vi "Dashboard Main.vi"(0 "Dashboard Tab":T1(tab)=enum."Custom") -> ()   [LabVIEW 2015]
uses:
  <vilib>/Utility/miscctls.llb/LVRowAndColumnTypeDef.ctl
  <vilib>/event_ctls.llb/eventvkey.ctl
  <vilib>/Rock Robotics/WPI/Dashboard/WPI_DashboardLogging Global.vi
  <vilib>/Rock Robotics/Network Tables/NT Read Numeric Array.vi
  <vilib>/Utility/config.llb/Write Key (String).vi
  <vilib>/Utility/config.llb/Write Key (I32).vi
  <vilib>/Utility/config.llb/NI_LVConfig.lvlib
panel:
  in  "TCP":refnum<k5>
  in  "Rec Mode":enum32{"Stop", "Record", "Playback"}(radio)
  in  "Vision":u16(ring) items=["Camera Off", "USB Camera SW", "USB Camera HW", "IP Camera"]
  out "Camera IP":string="172.22.11.2"
  out "Image Message":string="Timeout in Camera Communications"
  in  "Select Auto":string(combo)
  out "NT Connection":bool
  in  "Camera Settings":T2={"Frame Rate"=17, "Compression"=30, "Size"=1} {"Frame Rate" scale=1.0..30.0; "Size" items=["640x480", "320x240", "160x120"]}
  out "MotorChart R":cluster{"Numeric":dbl, "Numeric":dbl}(graph)
  out "MotorChart L":T3(graph)={"Numeric"=0.0, "Numeric"=0.0, "Battery V"=12.03125}
  out "MotorSliders R":cluster{"MotorSlide1":dbl, "MotorSlide2":dbl} {"MotorSlide2" scale=-1.0..1.0 scale format="%#_2e"; "MotorSlide1" scale=-1.0..1.0 scale format="%#_2e"}
  out "MotorSliders L":T4={"MotorSlide1"=0.0, "MotorSlide2"=0.0, "MotorSlide4 2"=12.03125} {"MotorSlide4 2" scale=0.0..14.0 scale format="%#_2e"; "MotorSlide2" scale=-1.0..1.0 scale format="%#_2e"; "MotorSlide1" scale=-1.0..1.0 scale format="%#_2e"}
  out "Gyro":dbl(knob) scale=0.0..360.0
  out "JS1 Z":dbl(slide) scale=-1.0..1.0 scale format="%#_2e"
  out "JS1 Graph":cluster{"X":dbl, "Y":dbl}[](graph)
  out "JS1 Buttons":T5
  out "JS2 Z":dbl(slide) scale=-1.0..1.0 scale format="%#_2e"
  out "JS2 Graph":cluster{"X":dbl, "Y":dbl}[](graph)
  out "JS2 Buttons":T5
  out "Mode":T6(ring)=enum."No Code"
  in  "DB Camera Config":bool
  out "fps":dbl format="%#.1g"
  out "Mbps":dbl format="%#.1g"
  out "Mbps LED":bool
  in  "DB/String 9":string
  in  "DB/String 8":string
  in  "DB/String 7":string
  in  "DB/String 6":string
  in  "DB/String 5":string
  in  "DB/String 4":string
  in  "DB/String 3":string
  in  "DB/String 2":string
  in  "DB/String 1":string
  in  "DB/String 0":string
  in  "DB/Slider 0":dbl(slide) scale=0.0..5.0
  in  "DB/Slider 1":dbl(slide) scale=0.0..5.0
  in  "DB/Slider 2":dbl(slide) scale=0.0..5.0
  in  "DB/Slider 3":dbl(slide) scale=0.0..5.0
  out "DB/LED 3":bool
  out "DB/LED 2":bool
  out "DB/LED 1":bool
  out "DB/LED 0":bool
  in  "DB/Button 3":bool
  in  "DB/Button 2":bool
  in  "DB/Button 1":bool
  in  "DB/Button 0":bool caption="New Name"
  in  "Left":bool
  out "Dist":dbl
  in  "Man_Cam":dbl
  out "Waveform Chart":cluster{"Numeric":dbl, "Numeric":dbl}(graph)
  in  "Shoot_Auto":bool
  in  "Auto":string(combo)
  in  "Delay_Auto":dbl(slide) scale=0.0..5.0
  in  "DB/MAO_Shooter":dbl
  in  "DB/Ramp_Rate":dbl=1.75
  in  "DB/FF_Gain":dbl=0.13
  in  "DB/I_Gain":dbl=1.0
  in  "DB/D_Gain":dbl
  in  "DB/P_Gain":dbl=0.03
  out "Angle_Error":dbl
  in  "En_Manual_Cam":bool
  in  "DB/Close":dbl=20.0
  in  "DB/Far_Cam":dbl=240.0
  in  "DB/Pitch_Dist":dbl=130.0
  in  "Right":bool
  in  "Test Slider":dbl(slide) scale=0.0..100.0 scale format="%#_3g"
  in  "On/Off":bool caption="Solenoid"
  in  "Test Name":u16(ring) items=["Select the test to run..."]
  in  "Test Tree":string(tree)
  in  "Motor":cluster{"Value":dbl, "Enable":bool} {"Value" scale=-1.0..1.0 scale format="%#_3g"}
  out "Progress":T7 {"Test Progress" scale=0.0..100.0}
  in  "Rev/Fwd":cluster{"Forward":bool, "Reverse":bool}
  in  "Test Ring":u16(ring) items=["Monochrome", "Color"]
  out "Cmd Status":string
  in  "Execute Command":bool
  in  "Command Params":string[][](table)
  in  "Command Selection":i32(listbox)
  in  "CheckList":i32(listbox)
  out "Tree":string(tree)
  out "Camera Image":T8(plugin-control)
  out "Background":bool
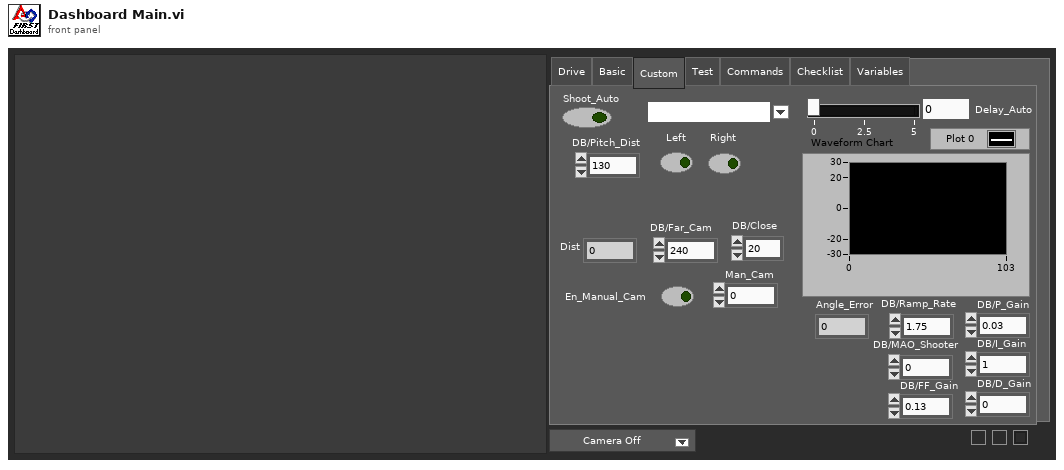
[diagram p1: front panel]
types:
  T1 = enum32{"Drive", "Basic", "Custom", "Test", "Commands", "Checklist", "Variables"}
  T2 = cluster{"Frame Rate":i32, "Compression":i32, "Size":u16}
  T3 = cluster{"Numeric":dbl, "Numeric":dbl, "Battery V":dbl}
  T4 = cluster{"MotorSlide1":dbl, "MotorSlide2":dbl, "MotorSlide4 2":dbl}
  T5 = cluster{bool, bool, bool, bool, bool, bool, bool, bool, bool, bool, bool, bool}
  T6 = enum8{"Tele-Op Disabled", "Tele-Op Enabled", "Auto Disabled", "Auto Enabled", "Test Disabled", "Test Enabled", "Disconnected", "No Code", "E-Stop"}
  T7 = cluster{"Test Progress":u8, "Test Progress Text":string}
  T8 = typedef "IMAQ Image.ctl" = refnum<image>
  T9 = cluster{"IDs":cluster{"RPC field ID":u16, "Unique ID":u16}, "String":string}
  T10 = enum32{"Drive", "Basic", "Custom", "Test", "Checklist", "Variables"}
  T11 = typedef "Image Type" = u32
  T12 = cluster{"Camera Image":refnum<vi>, "Dashboard Tab":refnum<vi>, "Background":refnum<vi>, "Vision":refnum<vi>, "Rec Mode":refnum<vi>, "Test Slider":refnum<vi>, "On/Off ":refnum<vi>, "Test Ring":refnum<vi>, "Rev/Fwd":refnum<vi>, "Test Name":refnum<vi>, "Motor":refnum<vi>, "Progress":refnum<vi>, "CheckList":refnum<vi>, "Tree":refnum<vi>, "Test Tree":refnum<vi>, "Command Params":refnum<vi>, "Command Selection":refnum<vi>, "Execute Command":refnum<vi>, "Cmd Status":refnum<vi>}
  T13 = cluster{"Error Strings":string, "Disable Counts":cluster{u16, u16}, "Rail Faults":cluster{u16, u16, u16}, "Robot IP":string, "DB Mode":u8, "Event Info":cluster{"Name":string, "Type":u8, "Number":u16, "Replay":u8}, "Camera Addr":string}
  T14 = cluster{"Storage":cluster{"Disk Free":u64, "RAM Block":u32, "RAM free":u32}, "CPU Utilization":cluster{"CPU % ISR":sgl, "CPU % Time Crit":sgl, "CPU % Timed Str":sgl, "CPU % High":sgl, "CPU % Above":sgl, "CPU % Normal":sgl, "CPU % Low":sgl}, "CAN":cluster{"% Bus Utilization":sgl, "Bus Off Cnt":u32, "TX_FIFO Full Cnt":u32, "Receive Error Cnt":u8, "Transmit Error Cnt":u8}, "HID":cluster{"HID Outputs":u32, "Rumble Low":u16, "Rumble High":u16}[]}
  T15 = cluster{"Status bits":cluster{"Test Mode":bool, "Autonomous":bool, "Enabled":bool, "Code Start":bool, "Brownout":bool, "Reserved 2":bool, "Reserved 3":bool, "E-Stop":bool}, "Code Trace":cluster{"Disabled":bool, "TeleOp":bool, "Auto":bool, "Test":bool}, "Controller Type":enum16{"unknown", "cRIO", "roboRio"}, "Code?":enum16{"unknown", "noCode", "code"}, "Battery V":dbl}
  T16 = cluster{"Control Bits":cluster{"TestMode":bool, "Autonomous":bool, "Enabled":bool, "FMS Present":bool, bool, bool, bool, "E-Stop":bool}, "Team Station ":u8, "Countdown":sgl, "Joystick Values":cluster{"Axes":dbl[], "Buttons":bool[], "POVs":i16[]}[]}
  T17 = cluster{"Axes":dbl[], "Buttons":bool[], "POVs":i16[]}[]
  T18 = cluster{"Axes":dbl[], "Buttons":bool[], "POVs":i16[]}
  T19 = cluster{"Buttons[0]":bool, "Buttons[1]":bool, "Buttons[2]":bool, "Buttons[3]":bool, "Buttons[4]":bool, "Buttons[5]":bool, "Buttons[6]":bool, "Buttons[7]":bool, "Buttons[8]":bool, "Buttons[9]":bool, "Buttons[10]":bool, "Buttons[11]":bool}
  T20 = typedef "NI_LVConfig.lvlib/Config Data RefNum.ctl" = refnum<k1>
  T21 = cluster{"Operation":enum16{"Update", "Clear"}, "Color Box":u32}[]
  T22 = typedef "eventvkey.ctl" = enum16{"ASCII", "Enter", "Return", "Shift", "Ctrl", "Alt", "Cmd", "Opt", "Caps", "NumLock", "Clear", "Break", "Up", "Down", "Left", "Right", "Insert", "Delete", "Home", "End", "PageUp", "PageDown", "Escape", "Help", "Pause", "ScrollLock", "F1", "F2", "F3", "F4", "F5", "F6", "F7", "F8", "F9", "F10", "F11", "F12", "F13", "F14", "F15", "F16", "F17", "F18", "F19", "F20", "F21", "F22", "F23", "F24", "Play", "VolumeUp", "VolumeDown", "Mute", "Two Byte Char"}
  T23 = cluster{"Image Size":bool, "Image Type":bool, "Pixel Value":bool, "ROI Information":bool, "Zoom Factor":bool}
  T24 = enum8{"Enabled", "Disabled", "Disabled and Grayed Out"}
  T25 = cluster{"Operation":enum16{"Update", "Clear"}, "Color Box":u32}
  T26 = typedef "LVRowAndColumnTypeDef.ctl" = cluster{"Row":i32, "Column":i32}
  T27 = cluster{"Shift":bool, "Ctrl":bool, "Alt":bool, "Cmd":bool, "Opt":bool}
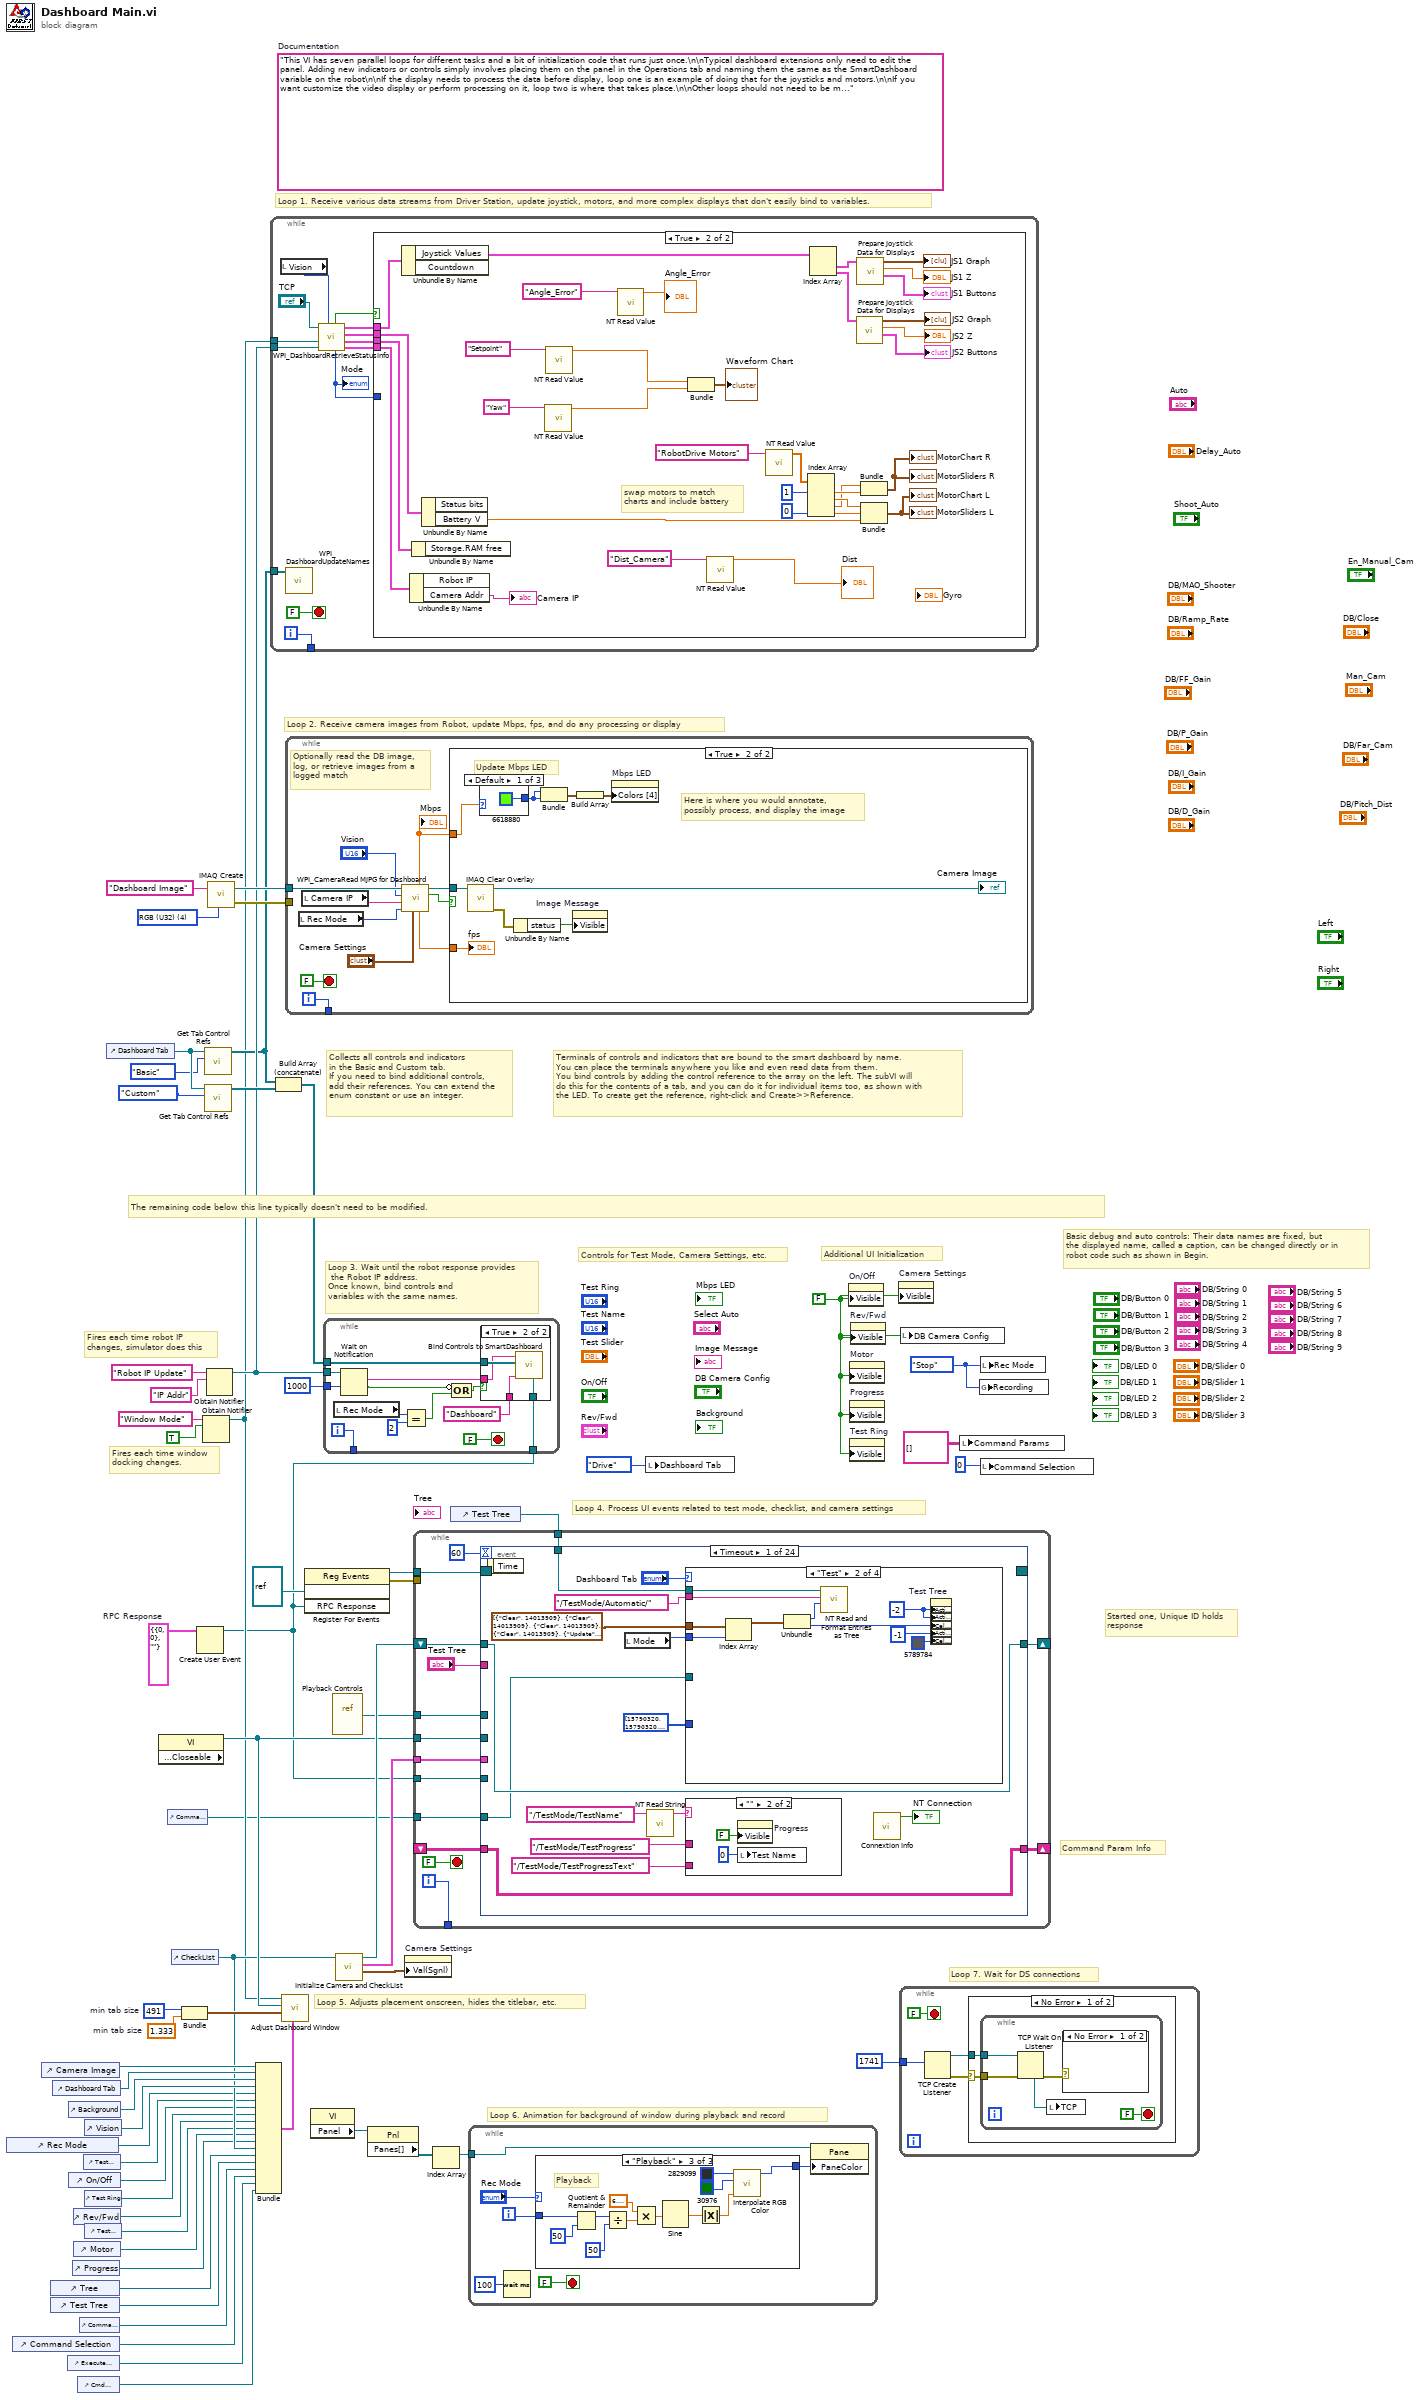
[diagram p0: block diagram]
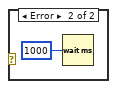
[diagram p2: hidden frame]
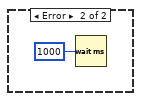
[diagram p3: hidden frame]
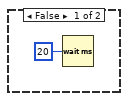
[diagram p4: hidden frame]
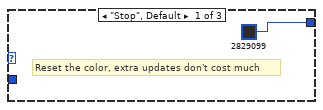
[diagram p5: hidden frame]
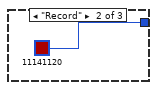
[diagram p6: hidden frame]
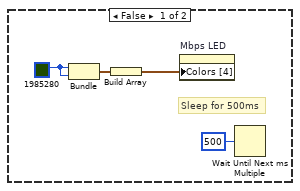
[diagram p8: hidden frame]
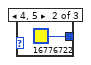
[diagram p9: hidden frame]
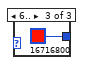
[diagram p10: hidden frame]
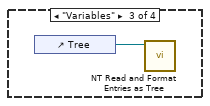
[diagram p12: hidden frame]
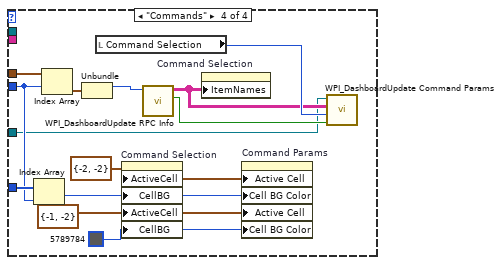
[diagram p13: hidden frame]
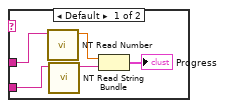
[diagram p14: hidden frame]
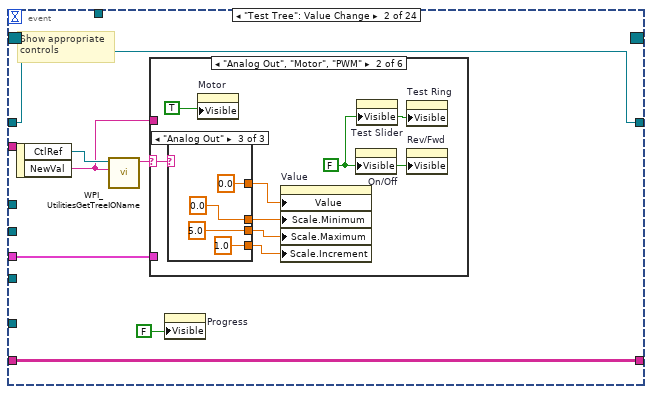
[diagram p15: hidden frame]
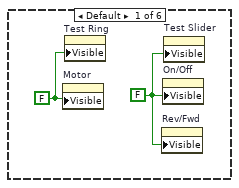
[diagram p16: hidden frame]
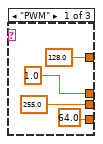
[diagram p17: hidden frame]
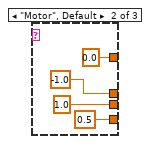
[diagram p18: hidden frame]
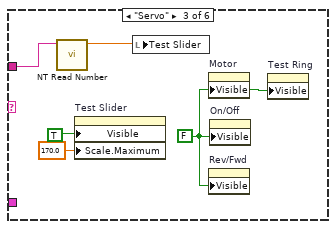
[diagram p19: hidden frame]
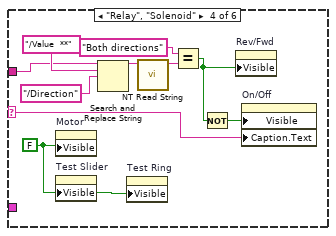
[diagram p20: hidden frame]
diagram:
  w7 = T9 {"IDs"={"RPC field ID"=0, "Unique ID"=0}, "String"=""}  # RPC Response
  w33 = 491  # min tab size
  w32 = 1.333  # min tab size
  w41 = enum32{"Stop", "Record", "Playback"}."Stop" ("Rec Mode")
  w15 = FALSE ("Visible")
  (unwired) "This VI has seven parallel loops for different tasks and a bit of initialization code that runs just once.\n\nTypical dashboard extensions only need to edit the panel. Adding new indicators or controls simply involves placing them on the panel in the Operations tab and naming them the same as the SmartDashboard variable on the robot\n\nIf the display needs to process the data before display, loop one is an example of doing that for the joysticks and motors.\n\nIf you want customize the video display or perform processing on it, loop two is where that takes place.\n\nOther loops should not need to be modified. They are pretty standard, and document the task they perform."  # Documentation
  w61 = T11 4 items=["Grayscale (U8)", "Grayscale (I16)", "Grayscale (SGL)", "Complex (CSG)", "RGB (U32)", "HSL (U32)", "RGB (U64)"] ("Image Type")
  # "Command Param Info"
  # "Started one, Unique ID holds\nresponse"
  # "Loop 7. Wait for DS connections"
  # "Basic debug and auto controls: Their data names are fixed, but\nthe displayed name, called a caption, can be changed directly or in\nrobot code such as shown in Begin."
  # "Controls for Test Mode, Camera Settings, etc."
  # "Additional UI Initialization"
  # "Loop 6. Animation for background of window during playback and record"
  # "Fires each time robot IP\nchanges, simulator does this"
  # "Fires each time window\ndocking changes."
  # "Collects all controls and indicators\nin the Basic and Custom tab.\nIf you need to bind additional controls,\nadd their references. You can extend the\nenum constant or use an integer."
  # "The remaining code below this line typically doesn't need to be modified."
  # "Loop 4. Process UI events related to test mode, checklist, and camera settings"
  # "Terminals of controls and indicators that are bound to the smart dashboard by name.\nYou can place the terminals anywhere you like and even read data from them.\nYou bind controls by adding the control reference to the array on the left. The subVI will\ndo this for the contents of a tab, and you can do it for individual items too, as shown with\nthe LED. To create get the reference, right-click and Create>>Reference."
  # "Loop 3. Wait until the robot response provides\n the Robot IP address.\nOnce known, bind controls and\nvariables with the same names."
  # "Loop 5. Adjusts placement onscreen, hides the titlebar, etc."
  # "Loop 1. Receive various data streams from Driver Station, update joystick, motors, and more complex displays that don't easily bind to variables."
  # "Loop 2. Receive camera images from Robot, update Mbps, fps, and do any processing or display"
  n1 = control-ref of="Rec Mode"() -> (w21:refnum<vi>)
  n2 = control-ref of="Command Selection"() -> (w6:refnum<vi>)
  n3 = control-ref of="Camera Image"() -> (w36:refnum<vi>)
  n4 = control-ref of="Tree"() -> (w25:refnum<vi>)
  n5 = control-ref of="Test Tree"() -> (w24:refnum<vi>)
  n6 = control-ref of="Dashboard Tab"() -> (w35:refnum<vi>)
  n7 = control-ref of="Execute Command"() -> (w8:refnum<vi>)
  n8 = control-ref of="Background"() -> (w30:refnum<vi>)
  n9 = control-ref of="On/Off"() -> (w19:refnum<vi>)
  n10 = control-ref of="Progress"() -> (w16:refnum<vi>)
  n11 = control-ref of="Rev/Fwd"() -> (w17:refnum<vi>)
  n12 = control-ref of="Motor"() -> (w22:refnum<vi>)
  n13 = control-ref of="Cmd Status"() -> (w2:refnum<vi>)
  n14 = control-ref of="Command Params"() -> (w9:refnum<vi>)
  n15 = control-ref of="Test Slider"() -> (w20:refnum<vi>)
  n16 = control-ref of="Vision"() -> (w34:refnum<vi>)
  n17 = control-ref of="Test Ring"() -> (w18:refnum<vi>)
  n18 = control-ref of="Test Name"() -> (w23:refnum<vi>)
  n19 = control-ref of="Dashboard Tab"() -> (w39:refnum<vi>)
  n20 = property class="VI" props=["Front Panel.Closeable"]() -> (reference out=w40:refnum<vi>)  [unwired: 2 in, 2 out]
  n21 = control-ref of="Command Params"() -> (w1:refnum<vi>)
  n22 = control-ref of="CheckList"() -> (w26:refnum<vi>)
  n23 = Bundle("min tab size"=w33, "min tab size"=w32) -> (w31:cluster{"min tab size":i32, "min tab size":dbl})  [unwired: 1 in]
  n24 = Create User Event(user event datatype=w7) -> (user event=w3:refnum<user-event>)  [unwired: 1 in, 1 out]
  n25 = Obtain Notifier(name (unnamed)="Window Mode", notification data type=TRUE) -> (notifier out=w12:refnum<notifier>)  [unwired: 2 in, 2 out]
  n26 = call <vilib>:"Get Tab Control Refs.vi"("Page Index"=T10."Basic" ("Dashboard Tab"), "TabControl in"=w39) -> ("ControlsOnPage"=w13:refnum<vi>[])  [unwired: 9 in]
  n27 = call <vilib>:"Get Tab Control Refs.vi"("Page Index"=T10."Custom" ("Dashboard Tab"), "TabControl in"=w39) -> ("ControlsOnPage"=w38:refnum<vi>[])  [unwired: 9 in]
  n28 = Obtain Notifier(name (unnamed)="Robot IP Update", notification data type="IP Addr" ("name (unnamed)")) -> (notifier out=w14:refnum<notifier>)  [unwired: 2 in, 2 out]
  n29 = call "IMAQ Create"("Image Name"="Dashboard Image", "Image Type"=w61) -> ("New Image"=w59:T8, "error out"=w58:errorcluster)  [unwired: 2 in, 1 out]
  n30 = Bundle("Camera Image"=w36, "Dashboard Tab"=w35, "Background"=w30, "Vision"=w34, "Rec Mode"=w21, "Test Slider"=w20, "On/Off"=w19, "Test Ring"=w18, "Rev/Fwd"=w17, "Test Name"=w23, "Motor"=w22, "Progress"=w16, "CheckList"=w26, "Tree"=w25, "Test Tree"=w24, "Command Params"=w9, "Command Selection"=w6, "Execute Command"=w8, "Cmd Status"=w2) -> (w27:T12)  [unwired: 1 in]
  n31 = while {
    tunnel: [w73] -> _
    tunnel: w14 -> [w67]
    tunnel: w13 -> [w66]
    tunnel: w12 -> [w62]
    i -> [w73]
    stop <- FALSE stop-if-true
    n32 = local read "Vision"() -> (w64:u16)
    n33 = call <vilib>:"WPI_DashboardUpdateNames.vi"("Controls on Tab"=w66) -> ()  [unwired: 11 in]
    n34 = call <vilib>:"WPI_DashboardRetrieveStatusInfo.vi"("Vision"=w64, "Binding Refnum"=w67, "Window Mode Notifier"=w62, "TCP Cnx"="TCP") -> ("Power and Errors"=w68:T13, "Robot Metrics"=w71:T14, "Status Info"=w72:T15, "Control Info"=w69:T16, "Robot Mode"=w65:T6, "Process?"=w70:bool)  [unwired: 2 in]
    "Mode" <- w65
    n35 = case shown="True" w70 {
      tunnel: w72 -> [_ w109]
      tunnel: w71 -> [_ w108]
      tunnel: w69 -> [_ w107]
      tunnel: w68 -> [_ w106]
      tunnel: w65 -> [_ _]
      frame False {
        n36 = Wait (ms)(milliseconds to wait=u32 20) -> ()  [unwired: 1 out]
      }
      frame True {
        # "swap motors to match\ncharts and include battery"
        n37 = Unbundle By Name(w107) -> ("Joystick Values"=w96:T17)  [unwired: 1 out]
        n38 = Unbundle By Name(w106) -> ("Camera Addr"=→"Camera IP":string)  [unwired: 1 out]
        n39 = Unbundle By Name(w108) -> ()  [unwired: 1 out]
        n40 = Unbundle By Name(w109) -> ("Battery V"=w97:dbl)  [unwired: 1 out]
        n41 = call-poly <vilib>:"NT Read Value.vi"("Name"="Yaw") -> ("Numeric"=w79:dbl)  [unwired: 9 in, 1 out]
        n42 = call-poly <vilib>:"NT Read Value.vi"("Name"="Setpoint") -> ("Numeric"=w80:dbl)  [unwired: 9 in, 1 out]
        n43 = call-poly <vilib>:"NT Read Value.vi"("Name"="Angle_Error") -> ("Numeric"=→"Angle_Error":dbl)  [unwired: 9 in, 1 out]
        n44 = Bundle("Numeric"=w80, "Numeric"=w79) -> (→"Waveform Chart":cluster{"Numeric":dbl, "Numeric":dbl})  [unwired: 1 in]
        n45 = call-poly <vilib>:"NT Read Value.vi"("Name"="Dist_Camera") -> ("Numeric"=→"Dist":dbl)  [unwired: 9 in, 1 out]
        n46 = call-poly <vilib>:"NT Read Value.vi"("Name"="RobotDrive Motors") -> ("Numeric Array"=w85:dbl[])  [unwired: 9 in, 1 out]
        n47 = Index Array(array=w85, index #1=1, index #4=0) -> (element #1=w101:dbl, element #2=w102:dbl, element #3=w100:dbl, element #4=w105:dbl)  [unwired: 2 in]
        n48 = Index Array(array=w96) -> (element #1=w95:T18, element #2=w90:T18)  [unwired: 2 in]
        n49 = call "Prepare Joystick Data for Displays.vi"("Joystick Values"=w90) -> ("Buttons"=→"JS2 Buttons":T19, "Z Axis"=→"JS2 Z":dbl, "Cartesian Data"=→"JS2 Graph":cluster{"X axis":dbl, "X axis":dbl}[])  [unwired: 8 in]
        n50 = call "Prepare Joystick Data for Displays.vi"("Joystick Values"=w95) -> ("Buttons"=→"JS1 Buttons":T19, "Z Axis"=→"JS1 Z":dbl, "Cartesian Data"=→"JS1 Graph":cluster{"X axis":dbl, "X axis":dbl}[])  [unwired: 8 in]
        n51 = Bundle("Numeric"=w100, "Numeric"=w101) -> (→"MotorChart R" →"MotorSliders R":cluster{"Numeric":dbl, "Numeric":dbl})  [unwired: 1 in]
        n52 = Bundle("Numeric"=w102, "Numeric"=w105, "Battery V"=w97) -> (→"MotorChart L" →"MotorSliders L":T3)  [unwired: 1 in]
      }
    }
  }
  n53 = Build Array (concatenate)(w13, w38) -> (w37:refnum<vi>[])
  n54 = call "Adjust Dashboard Window.vi"("Sizing Refnums"=w27, "Size Constraints"=w31, "VI"=w40, "WIn Mode"=w12) -> ()  [unwired: 8 in]
  n55 = while {
    tunnel: w59 -> [w118]
    tunnel: w58 -> [_]
    tunnel: [w119] -> _
    i -> [w119]
    stop <- FALSE stop-if-true
    # "Optionally read the DB image,\nlog, or retrieve images from a\nlogged match"
    n56 = local read "Rec Mode"() -> (w113:enum32{"Stop", "Record", "Playback"})
    n57 = local read "Camera IP"() -> (w111:string)
    n58 = call <vilib>:"WPI_CameraRead MJPG for Dashboard.vi"("Camera Settings"="Camera Settings", "Rec Mode"=w113, "Camera IP"=w111, "Camera Mode"="Vision", "Refnum in"=w118) -> ("Active"=w116:bool, "Refnum out"=w117:T8, "FPS"=w115:dbl, "Bandwidth (Mbps)"=w110:dbl)  [unwired: 3 in]
    "Mbps" <- w110
    n59 = case shown="True" w116 {
      tunnel: w117 -> [_ w128]
      tunnel: w110 -> [_ w127]
      tunnel: w115 -> [_ w125]
      frame False {
        w121 = u32 1985280 ("Color Box")
        # "Sleep for 500ms"
        n60 = Bundle("Color Box"=w121, "Color Box"=w121) -> (w123:cluster{"Color Box":u32, "Color Box":u32})  [unwired: 1 out]
        n61 = Build Array(w123) -> (w122:cluster{"Color Box":u32, "Color Box":u32}[])
        n62 = property on="Mbps LED" class="Bool (strict)"("Colors [4]"=w122) -> ()  [unwired: 2 in, 2 out]
        n63 = Wait Until Next ms Multiple(millisecond multiple=u32 500) -> ()  [unwired: 1 out]
      }
      frame True {
        # "Here is where you would annotate,\npossibly process, and display the image"
        # "Update Mbps LED"
        n64 = call "IMAQ Clear Overlay"("Image"=w128) -> ("error out"=w132:errorcluster, "Image Out"=→"Camera Image":T8)  [unwired: 2 in, 7 out]
        n65 = case shown="Default" w127 {
          tunnel: [u32 6618880 ("Color Box") u32 16776722 ("Color Box") u32 16716800 ("Color Box")] -> w129
          frame Default {
          }
          frame 4, 5 {
          }
          frame 6.. {
          }
        }
        n66 = Unbundle By Name(w132) -> ("status"=w133:bool)
        n67 = Bundle("Color Box"=w129, "Color Box"=w129) -> (w131:cluster{"Color Box":u32, "Color Box":u32})  [unwired: 1 out]
        n68 = property on="Image Message" class="Str"("Visible"=w133) -> ()  [unwired: 2 in, 2 out]
        n69 = Build Array(w131) -> (w130:cluster{"Color Box":u32, "Color Box":u32}[])
        n70 = property on="Mbps LED" class="Bool (strict)"("Colors [4]"=w130) -> ()  [unwired: 2 in, 2 out]
        "fps" <- w125
      }
    }
  }
  n71 = register-events(refnum<vi> refnum, w3) -> (reference out=w45:refnum<event-registration>, error out=w44:errorcluster)  [unwired: 2 in]
  n72 = property class="VI"() -> ("Panel"=w48:refnum<vi>)  [unwired: 2 in, 2 out]
  n73 = while {
    tunnel: w37 -> [w149]
    tunnel: w14 -> [w147]
    tunnel: [w145] -> _
    tunnel: u32 1000 ("milliseconds to wait") -> [w144]
    tunnel: w3 -> [w137]
    i -> [w145]
    stop <- FALSE stop-if-true
    n74 = local read "Rec Mode"() -> (w140:enum32{"Stop", "Record", "Playback"})
    n75 = Wait on Notification(notifier=w147, timeout in ms (-1)=w144) -> (notification=w146:string, timed out?=w142:bool)  [unwired: 2 in, 2 out]
    n76 = Equal?(x=w140, y=u16 2 ("Rec Mode")) -> (x = y?=w141:bool)
    n77 = Compound Arithmetic op=OR(invert w142, w141) -> (w143:bool)
    n78 = case shown="True" w143 {
      tunnel: w149 -> [_ w153]
      tunnel: w146 -> [_ w152]
      tunnel: "Dashboard" -> [_ w151]
      tunnel: w137 -> [_ w150]
      frame False {
      }
      frame True {
        n79 = call <vilib>:"Bind Controls to SmartDashboard.vi"("RPC ref"=w150, "Client Name"=w151, "Bound Control Refs"=w153, "Server IP Address"=w152) -> ()  [unwired: 8 in]
      }
    }
  }
  n80 = vi-ref "Playback Controls.vi"() -> (w46:refnum<vi>)
  n81 = call "Initialize Camera and CheckList.vi"("ListBox in"=w26) -> ("Cluster"=w52:cluster{"value":i32, "value":i32, "index":i32}, "Array"=w53:cluster{string[]}[], "File Refnum"=w51:T20)  [unwired: 8 in]
  n82 = property class="Pnl"(reference=w48) -> ("Panes[]"=w49:refnum<vi>[])  [unwired: 1 in, 2 out]
  n83 = property on="Camera Settings" class="Clust (strict)"("Val(Sgnl)"=w52) -> ()  [unwired: 2 in, 2 out]
  n84 = Index Array(array=w49) -> (element=w47:refnum<vi>)  [unwired: 1 in]
  n85 = control-ref of="Test Tree"() -> (w50:refnum<vi>)
  n86 = while {
    tunnel: w53 -> [w165]
    shift-right: [w164] -> _
    shift-left: w51 -> [w163]
    tunnel: [w162] -> _
    tunnel: w50 -> [w161]
    tunnel: w46 -> [w160]
    tunnel: w45 -> [w159]
    tunnel: w44 -> [_]
    tunnel: w40 -> [w158]
    tunnel: w3 -> [w157]
    tunnel: w1 -> [w156]
    shift-right: [w155] -> _
    shift-left: _ -> [w154]
    i -> [w162]
    stop <- FALSE stop-if-true
    n87 = event shown="[0] Timeout" {
      selector: w159 -> [_ _ _ _ _ _ _ _ _ _ _ _ _ _ _ _ _ _ _ _ _ _ _ _]
      dyn-events: [_ _ _ _ _ _ _ _ _ _ _ _ _ _ _ _ _ _ w474 _ _ _ _ _] -> _
      timeout: u32 60 ("milliseconds to wait") -> [_ _ _ _ _ _ _ _ _ _ _ _ _ _ _ _ _ _ _ _ _ _ _ _]
      tunnel: w161 -> [w178 _ _ _ _ _ _ _ _ _ _ _ _ _ _ _ _ _ _ _ _ _ _ _]
      tunnel: "Test Tree" -> [_ _ _ _ _ _ _ _ _ _ _ _ _ w437 w446 w449 w454 w463 _ _ _ _ _ _]
      tunnel: w165 -> [_ w216 _ _ _ _ _ _ _ _ _ w399 w430 _ _ _ _ _ _ _ _ _ _ _]
      tunnel: [w175 w215 w319 w325 w335 w339 w345 w357 w365 w371 w384 w398 w423 w436 w444 w448 w453 w462 w476 w492 w494 w502 w513 w518] -> w164
      tunnel: w163 -> [w175 w215 w319 w325 w335 w339 w345 w357 w365 w371 w384 w397 w423 w436 w444 w448 w453 w462 w476 w492 w494 w502 w513 w518]
      tunnel: w160 -> [_ _ _ _ _ _ _ _ _ _ _ _ _ _ _ _ _ _ w477 _ w497 _ _ _]
      tunnel: w158 -> [_ _ _ _ _ _ _ _ _ _ _ _ _ _ _ _ _ _ w472 _ _ _ _ _]
      tunnel: w157 -> [_ _ _ _ _ _ _ _ _ _ _ _ _ _ _ _ _ _ w468 _ _ _ _ _]
      tunnel: w156 -> [w170 _ _ _ _ _ w343 _ _ _ _ _ _ _ _ _ _ _ _ _ _ _ _ _]
      tunnel: [w169 w214 w318 w324 w334 w340 w341 w351 w362 w370 w383 w396 w422 w435 w443 w447 w452 w461 w467 w490 w493 w498 w506 w519] -> w155
      tunnel: w154 -> [w169 w214 w318 w324 w334 w340 w341 _ _ w370 w383 w396 w422 w435 w443 w447 w452 w461 w467 w490 w493 w498 w506 w519]
      event Timeout {
        n88 = event-data() -> ()  [unwired: 1 in, 1 out]
        n89 = local read "Mode"() -> (w172:T6)
        n90 = call <vilib>:"NT Read String.vi"("Name"="/TestMode/TestName") -> ("String"=w181:string)  [unwired: 9 in, 1 out]
        n91 = case shown="\"Test\"" "Dashboard Tab" {
          tunnel: w178 -> [_ w192 _ _]
          tunnel: "/TestMode/Automatic/" ("Name Pattern") -> [_ w191 _ _]
          tunnel: T21 [{"Operation"=enum."Clear", "Color Box"=14013909}, {"Operation"=enum."Clear", "Color Box"=14013909}, {"Operation"=enum."Clear", "Color Box"=14013909}, {"Operation"=enum."Clear", "Color Box"=14013909}, {"Operation"=enum."Update", "Color Box"=14013909}, {"Operation"=enum."Update", "Color Box"=16777215}, {"Operation"=enum."Clear", "Color Box"=14013909}, {"Operation"=enum."Clear", "Color Box"=14013909}, {"Operation"=enum."Clear", "Color Box"=14013909}] -> [_ w184 _ w201]
          tunnel: w172 -> [_ w183 _ w200]
          tunnel: u32[] [15790320, 15790320, 15790320, 15790320, 16777215, 16777215, 15790320, 15790320, 15790320] -> [_ _ _ w206]
          tunnel: w170 -> [_ _ _ w194]
          frame "Custom", Default {
          }
          frame "Test" {
            w190 = -2 ("Active Item:Row Number")
            n92 = Index Array(array=w184, index=w183) -> (element=w185:T25)
            n93 = Unbundle(w185) -> ("Operation"=w186:enum16{"Update", "Clear"}, "Color Box"=w187:u32)
            n94 = call <vilib>:"NT Read and Format Entries as Tree.vi"("Operation"=w186, "Name Pattern"=w191, "Tree Refnum"=w192) -> ()  [unwired: 7 in, 2 out]
            n95 = property on="Test Tree" class="Tree (strict)"("Active Item Row Number"=w190, "ActiveColNum"=w190, "CellBG"=w187, "Active Item Row Number"=-1 ("Active Item:Row Number"), "CellBG"=u32 5789784 ("Color Box")) -> ()  [unwired: 2 in, 2 out]
          }
          frame "Variables" {
            n96 = control-ref of="Tree"() -> (w193:refnum<vi>)
            n97 = call <vilib>:"NT Read and Format Entries as Tree.vi"("Tree Refnum"=w193) -> ()  [unwired: 9 in, 2 out]
          }
          frame "Commands" {
            w202 = u32 5789784 ("Color Box")
            w203 = T26 {"Row"=-1, "Column"=-2} ("Active Cell:Active Cell")
            w205 = T26 {"Row"=-2, "Column"=-2} ("Active Cell:Active Cell")
            n98 = Index Array(array=w206, index=w200) -> (element=w204:u32)
            n99 = Index Array(array=w201, index=w200) -> (element=w199:T25)
            n100 = Unbundle(w199) -> ("Operation"=w198:enum16{"Update", "Clear"})  [unwired: 1 out]
            n101 = local read "Command Selection"() -> (w197:i32)
            n102 = property on="Command Selection" class="MCListbox (strict)"("ActiveCell"=w205, "CellBG"=w204, "ActiveCell"=w203, "CellBG"=w202) -> ()  [unwired: 2 in, 2 out]
            n103 = call <vilib>:"WPI_DashboardUpdate RPC Info.vi"("Operation"=w198) -> ("update"=w196:bool, "commands"=w195:string[][])  [unwired: 9 in]
            n104 = property on="Command Selection" class="MCListbox (strict)"("ItemNames"=w195) -> ()  [unwired: 2 in, 2 out]
            n105 = property on="Command Params" class="Tbl (strict)"("Active Cell"=w205, "Cell BG Color"=w204, "Active Cell"=w203, "Cell BG Color"=w202) -> ()  [unwired: 2 in, 2 out]
            n106 = call <vilib>:"WPI_DashboardUpdate Command Params.vi"("Update"=w196, "NewVal"=w197, "Commands"=w195, "Param Tbl"=w194) -> ()  [unwired: 7 in, 1 out]
          }
        }
        n107 = case shown="\"\"" w181 {
          tunnel: "/TestMode/TestProgress" ("Name") -> [w208 _]
          tunnel: "/TestMode/TestProgressText" ("Name") -> [w207 _]
          frame Default {
            n108 = call <vilib>:"NT Read Number.vi"("Name"=w208) -> ("Numeric"=w209:dbl)  [unwired: 9 in, 1 out]
            n109 = call <vilib>:"NT Read String.vi"("Name"=w207) -> ("String"=w210:string)  [unwired: 9 in, 1 out]
            n110 = Bundle("Numeric"=w209, "String"=w210) -> (→"Progress":cluster{"Numeric":dbl, "String":string})  [unwired: 1 in]
          }
          frame "" {
            n111 = property on="Progress" class="Clust (strict)"("Visible"=FALSE) -> ()  [unwired: 2 in, 2 out]
            n112 = local write "Test Name"(u16 0) -> ()
          }
        }
        n113 = call <vilib>:"Connextion Info.vi"() -> ("Connected"=→"NT Connection":bool)  [unwired: 10 in, 1 out]
      }
      event "Test Tree": Value Change {
        # "Show appropriate\ncontrols"
        n114 = event-data() -> ("CtlRef"=w219:refnum<vi>, "NewVal"=w217:string)  [unwired: 1 in]
        n115 = call <vilib>:"WPI_UtilitiesGetTreeIOName.vi"("NewVal"=w217, "TreeControl in"=w219) -> ("I/O Name"=w220:string)  [unwired: 9 in]
        n116 = case shown="\"Analog Out\", \"Motor\", \"PWM\"" w220 {
          selector: w220 -> [_ w227 _ w249 w258 _]
          tunnel: w217 -> [_ _ w246 w248 _ w265]
          tunnel: w216 -> [_ _ _ _ _ w264]
          frame Default {
            w222 = FALSE ("Visible")
            w221 = FALSE ("Visible")
            n117 = property on="Motor" class="Clust (strict)"("Visible"=w221) -> ()  [unwired: 2 in, 2 out]
            n118 = property on="Test Ring" class="Ring (strict)"("Visible"=w221) -> ()  [unwired: 2 in, 2 out]
            n119 = property on="Rev/Fwd" class="Clust (strict)"("Visible"=w222) -> ()  [unwired: 2 in, 2 out]
            n120 = property on="On/Off" class="Bool (strict)"("Visible"=w222) -> ()  [unwired: 2 in, 2 out]
            n121 = property on="Test Slider" class="Slide (strict)"("Visible"=w222) -> ()  [unwired: 2 in, 2 out]
          }
          frame "Analog Out", "Motor", "PWM" {
            w228 = FALSE ("Visible")
            n122 = case shown="\"Analog Out\"" w227 {
              tunnel: [1.0 ("Value") -1.0 ("Value") 0.0 ("Value")] -> w226
              tunnel: [255.0 ("Value") 1.0 ("Value") 5.0 ("Value")] -> w225
              tunnel: [128.0 ("Value") 0.0 ("Value") 0.0 ("Value")] -> w224
              tunnel: [64.0 ("Value") 0.5 ("Value") 1.0 ("Value")] -> w223
              frame "PWM" {
              }
              frame "Motor", Default {
              }
              frame "Analog Out" {
              }
            }
            n123 = property on="Motor" class="Clust (strict)"("Visible"=TRUE) -> ()  [unwired: 2 in, 2 out]
            n124 = property on="Value" class="Slide (strict)"("Value"=w224, "Scale.Minimum"=w226, "Scale.Maximum"=w225, "Scale.Increment"=w223) -> ()  [unwired: 2 in, 2 out]
            n125 = property on="On/Off" class="Bool (strict)"("Visible"=w228) -> ()  [unwired: 2 in, 2 out]
            n126 = property on="Test Slider" class="Slide (strict)"("Visible"=w228) -> ()  [unwired: 2 in, 2 out]
            n127 = property on="Test Ring" class="Ring (strict)"("Visible"=w228) -> ()  [unwired: 2 in, 2 out]
            n128 = property on="Rev/Fwd" class="Clust (strict)"("Visible"=w228) -> ()  [unwired: 2 in, 2 out]
          }
          frame "Servo" {
            w244 = FALSE ("Visible")
            n129 = call <vilib>:"NT Read Number.vi"("Name"=w246) -> ("Numeric"=w245:dbl)  [unwired: 9 in, 1 out]
            n130 = property on="Test Slider" class="Slide (strict)"("Visible"=TRUE, "Scale.Maximum"=170.0 ("Scale.Range:Maximum")) -> ()  [unwired: 2 in, 2 out]
            n131 = local write "Test Slider"(w245) -> ()
            n132 = property on="Motor" class="Clust (strict)"("Visible"=w244) -> ()  [unwired: 2 in, 2 out]
            n133 = property on="Rev/Fwd" class="Clust (strict)"("Visible"=w244) -> ()  [unwired: 2 in, 2 out]
            n134 = property on="On/Off" class="Bool (strict)"("Visible"=w244) -> ()  [unwired: 2 in, 2 out]
            n135 = property on="Test Ring" class="Ring (strict)"("Visible"=w244) -> ()  [unwired: 2 in, 2 out]
          }
          frame "Relay", "Solenoid" {
            w247 = FALSE ("Visible")
            n136 = property on="Motor" class="Clust (strict)"("Visible"=w247) -> ()  [unwired: 2 in, 2 out]
            n137 = property on="Test Slider" class="Slide (strict)"("Visible"=w247) -> ()  [unwired: 2 in, 2 out]
            n138 = Search and Replace String(input string=w248, search string="/Value  **", replace string="/Direction") -> (result string=w254:string)  [unwired: 5 in, 3 out]
            n139 = property on="Test Ring" class="Ring (strict)"("Visible"=w247) -> ()  [unwired: 2 in, 2 out]
            n140 = call <vilib>:"NT Read String.vi"("Name"=w254) -> ("String"=w252:string)  [unwired: 9 in, 1 out]
            n141 = Equal?(x="Both directions", y=w252) -> (x = y?=w250:bool)
            n142 = Not(x=w250) -> (.not. x?=w251:bool)
            n143 = property on="Rev/Fwd" class="Clust (strict)"("Visible"=w250) -> ()  [unwired: 2 in, 2 out]
            n144 = property on="On/Off" class="Bool (strict)"("Visible"=w251, "Caption.Text"=w249) -> ()  [unwired: 2 in, 2 out]
          }
          frame "Compressor", "Digital Out" {
            w257 = FALSE ("Visible")
            # "Get direction and finish"
            n145 = property on="Motor" class="Clust (strict)"("Visible"=w257) -> ()  [unwired: 2 in, 2 out]
            n146 = property on="Test Slider" class="Slide (strict)"("Visible"=w257) -> ()  [unwired: 2 in, 2 out]
            n147 = property on="Test Ring" class="Ring (strict)"("Visible"=w257) -> ()  [unwired: 2 in, 2 out]
            n148 = property on="On/Off" class="Bool (strict)"("Visible"=TRUE, "Caption.Text"=w258) -> ()  [unwired: 2 in, 2 out]
            n149 = property on="Rev/Fwd" class="Clust (strict)"("Visible"=FALSE) -> ()  [unwired: 2 in, 2 out]
          }
          frame "Camera" {
            n150 = call <vilib>:"Get Last Path Segment.vi"("String in"=w265) -> ("String out"=w266:string)  [unwired: 10 in]
            n151 = property on="On/Off" class="Bool (strict)"("Visible"=FALSE) -> ()  [unwired: 2 in, 2 out]
            n152 = property on="Motor" class="Clust (strict)"("Visible"=FALSE) -> ()  [unwired: 2 in, 2 out]
            n153 = property on="Rev/Fwd" class="Clust (strict)"("Visible"=FALSE) -> ()  [unwired: 2 in, 2 out]
            n154 = case shown="\"White Balance  **\"" w266 {
              tunnel: w265 -> [w272 w281 w290 w299 w308 _ w314]
              tunnel: w264 -> [w270 w278 w287 w296 w305 _ _]
              frame "Size  **" {
                n155 = Index Array(array=w270) -> (element=w269:cluster{string[]})  [unwired: 1 in]
                n156 = call <vilib>:"NT Read String.vi"("Name"=w272) -> ("String"=w271:string)  [unwired: 9 in, 1 out]
                n157 = Unbundle(w269) -> (w267:string[])
                n158 = Match First String(2:w267, 3:w271) -> (0:w268:i32)  [unwired: 1 out]
                n159 = property on="Test Ring" class="Ring (strict)"("Value"=w268, "Strings []"=w267) -> ()  [unwired: 2 in, 2 out]
                n160 = property on="Test Ring" class="Ring (strict)"("Visible"=TRUE) -> ()  [unwired: 2 in, 2 out]
                n161 = property on="Test Slider" class="Slide (strict)"("Visible"=FALSE) -> ()  [unwired: 2 in, 2 out]
              }
              frame "White Balance  **" {
                n162 = Index Array(array=w278, index=1) -> (element=w279:cluster{string[]})
                n163 = call <vilib>:"NT Read String.vi"("Name"=w281) -> ("String"=w280:string)  [unwired: 9 in, 1 out]
                n164 = Unbundle(w279) -> (w276:string[])
                n165 = Match First String(2:w276, 3:w280) -> (0:w275:i32)  [unwired: 1 out]
                n166 = property on="Test Ring" class="Ring (strict)"("Value"=w275, "Strings []"=w276) -> ()  [unwired: 2 in, 2 out]
                n167 = property on="Test Ring" class="Ring (strict)"("Visible"=TRUE) -> ()  [unwired: 2 in, 2 out]
                n168 = property on="Test Slider" class="Slide (strict)"("Visible"=FALSE) -> ()  [unwired: 2 in, 2 out]
              }
              frame "Exposure  **" {
                n169 = Index Array(array=w287, index=2) -> (element=w288:cluster{string[]})
                n170 = call <vilib>:"NT Read String.vi"("Name"=w290) -> ("String"=w289:string)  [unwired: 9 in, 1 out]
                n171 = Unbundle(w288) -> (w284:string[])
                n172 = Match First String(2:w284, 3:w289) -> (0:w285:i32)  [unwired: 1 out]
                n173 = property on="Test Ring" class="Ring (strict)"("Value"=w285, "Strings []"=w284) -> ()  [unwired: 2 in, 2 out]
                n174 = property on="Test Ring" class="Ring (strict)"("Visible"=TRUE) -> ()  [unwired: 2 in, 2 out]
                n175 = property on="Test Slider" class="Slide (strict)"("Visible"=FALSE) -> ()  [unwired: 2 in, 2 out]
              }
              frame "Exposure Priority  **" {
                n176 = Index Array(array=w296, index=3) -> (element=w297:cluster{string[]})
                n177 = call <vilib>:"NT Read String.vi"("Name"=w299) -> ("String"=w298:string)  [unwired: 9 in, 1 out]
                n178 = Unbundle(w297) -> (w293:string[])
                n179 = Match First String(2:w293, 3:w298) -> (0:w294:i32)  [unwired: 1 out]
                n180 = property on="Test Ring" class="Ring (strict)"("Value"=w294, "Strings []"=w293) -> ()  [unwired: 2 in, 2 out]
                n181 = property on="Test Ring" class="Ring (strict)"("Visible"=TRUE) -> ()  [unwired: 2 in, 2 out]
                n182 = property on="Test Slider" class="Slide (strict)"("Visible"=FALSE) -> ()  [unwired: 2 in, 2 out]
              }
              frame "Color Enable  **" {
                n183 = Index Array(array=w305, index=4) -> (element=w306:cluster{string[]})
                n184 = call <vilib>:"NT Read String.vi"("Name"=w308) -> ("String"=w307:string)  [unwired: 9 in, 1 out]
                n185 = Unbundle(w306) -> (w302:string[])
                n186 = Match First String(2:w302, 3:w307) -> (0:w303:i32)  [unwired: 1 out]
                n187 = property on="Test Ring" class="Ring (strict)"("Value"=w303, "Strings []"=w302) -> ()  [unwired: 2 in, 2 out]
                n188 = property on="Test Ring" class="Ring (strict)"("Visible"=TRUE) -> ()  [unwired: 2 in, 2 out]
                n189 = property on="Test Slider" class="Slide (strict)"("Visible"=FALSE) -> ()  [unwired: 2 in, 2 out]
              }
              frame Default {
                n190 = property on="Test Ring" class="Ring (strict)"("Visible"=FALSE) -> ()  [unwired: 2 in, 2 out]
                n191 = property on="Test Slider" class="Slide (strict)"("Visible"=FALSE) -> ()  [unwired: 2 in, 2 out]
              }
              frame "Brightness  **", "Color Level  **", "Compression  **", "FPS  **", "Sharpness  **" {
                n192 = call <vilib>:"NT Read Number.vi"("Name"=w314) -> ("Numeric"=w313:dbl)  [unwired: 9 in, 1 out]
                n193 = local write "Test Slider"(w313) -> ()
                n194 = property on="Test Slider" class="Slide (strict)"("Visible"=TRUE, "Scale.Maximum"=100.0 ("Scale.Range:Maximum")) -> ()  [unwired: 2 in, 2 out]
                n195 = property on="Test Ring" class="Ring (strict)"("Visible"=FALSE) -> ()  [unwired: 2 in, 2 out]
              }
            }
          }
        }
        n196 = property on="Progress" class="Clust (strict)"("Visible"=FALSE) -> ()  [unwired: 2 in, 2 out]
      }
      event "Test Name": Mouse Enter {
        # "Populate the ring with the list of tests"
        n197 = event-data() -> ()  [unwired: 1 in, 1 out]
        n198 = call <vilib>:"NT Read String Array.vi"("Name"="/TestMode/TestList") -> ("String Array"=w323:string[])  [unwired: 9 in, 1 out]
        n199 = Build Array (concatenate)("Select the test to run...", w323) -> (w322:string[])
        n200 = property on="Test Name" class="Ring (strict)"("Strings []"=w322) -> ()  [unwired: 2 in, 2 out]
      }
      event "Test Name": Value Change {
        w326 = FALSE ("Visible")
        # "Tell the robot the test name to run"
        n201 = event-data() -> ("NewVal"=w330:u16)  [unwired: 1 in]
        n202 = property on="Test Name" class="Ring (strict)"() -> ("Strings []"=w331:string[])  [unwired: 2 in, 2 out]
        n203 = local write "Progress"(T7 {"Test Progress"=0, "Test Progress Text"=""} ("Progress")) -> ()
        n204 = Index Array(array=w331, index=w330) -> (element=w329:string)
        n205 = call <vilib>:"NT Write String.vi"("String"=w329, "Name"="/TestMode/TestName") -> ()  [unwired: 9 in, 1 out]
        n206 = property on="Progress" class="Clust (strict)"("Visible"=TRUE) -> ()  [unwired: 2 in, 2 out]
        n207 = property on="Motor" class="Clust (strict)"("Visible"=w326) -> ()  [unwired: 2 in, 2 out]
        n208 = property on="Test Slider" class="Slide (strict)"("Visible"=w326) -> ()  [unwired: 2 in, 2 out]
        n209 = property on="On/Off" class="Bool (strict)"("Visible"=w326) -> ()  [unwired: 2 in, 2 out]
        n210 = property on="Rev/Fwd" class="Clust (strict)"("Visible"=w326) -> ()  [unwired: 2 in, 2 out]
        n211 = property on="Test Ring" class="Ring (strict)"("Visible"=w326) -> ()  [unwired: 2 in, 2 out]
      }
      event "Select Auto": Mouse Enter {
        # "Populate the combo box with the list of autonomous options"
        n212 = event-data() -> ()  [unwired: 1 in, 1 out]
        n213 = call <vilib>:"NT Read String Array.vi"("Name"="Auto List") -> ("String Array"=w333:string[])  [unwired: 9 in, 1 out]
        n214 = property on="Select Auto" class="CmbBox"("Strings[]"=w333) -> ()  [unwired: 2 in, 2 out]
      }
      event "Select Auto": Value Change {
        # "User modified the Auto Selection. Write to NT variable so robot knows."
        n215 = event-data() -> ("NewVal"=w337:string)  [unwired: 1 in]
        n216 = call <vilib>:"NT Write String.vi"("String"=w337, "Name"="Auto Selector") -> ()  [unwired: 9 in, 1 out]
      }
      event "Command Selection": Value Change {
        # "Get the params and show in table"
        n217 = event-data() -> ("NewVal"=w344:i32)  [unwired: 1 in]
        n218 = property on="Command Selection" class="MCListbox (strict)"() -> ("ItemNames"=w342:string[][])  [unwired: 2 in, 2 out]
        n219 = call <vilib>:"WPI_DashboardUpdate Command Params.vi"("NewVal"=w344, "Commands"=w342, "Param Tbl"=w343) -> ()  [unwired: 8 in, 1 out]
      }
      event "Execute Command": Value Change {
        # "Started one, Unique ID holds\nresponse"
        n220 = event-data() -> ()  [unwired: 1 in, 1 out]
        n221 = property on="Command Selection" class="MCListbox (strict)"() -> ("ItemNames"=w356:string[][])  [unwired: 2 in, 2 out]
        n222 = Index Array(array=w356, index (row)="Command Selection", index (col)=0) -> (element=w354:string)
        n223 = call <vilib>:"Invoke Commands.vi"("Command Params"="Command Params", "Function Name"=w354) -> ("Params"=w350:u8, "Started"=w349:bool)  [unwired: 7 in, 1 out]
        n224 = Array Subset(array="Command Params", length (row)=w350) -> (w351:string[][])  [unwired: 3 in]
        n225 = Select(t="Executing" ("Cmd Status"), s=w349, f="" ("Cmd Status")) -> (s? t:f=→"Cmd Status":string)
      }
      event "Command Selection": Double Click {
        n226 = event-data() -> ("Row"=w366:i32)  [unwired: 1 in]
        n227 = property on="Command Selection" class="MCListbox (strict)"() -> ("ItemNames"=w369:string[][])  [unwired: 2 in, 2 out]
        n228 = local read "Command Params"() -> (w364:string[][])
        n229 = Index Array(array=w369, index (row)=w366, index (col)=0) -> (element=w367:string)
        n230 = call <vilib>:"Invoke Commands.vi"("Command Params"=w364, "Function Name"=w367) -> ("Params"=w363:u8, "Started"=w358:bool)  [unwired: 7 in, 1 out]
        n231 = Array Subset(array=w364, length (row)=w363) -> (w362:string[][])  [unwired: 3 in]
        n232 = Select(t="Executing" ("Cmd Status"), s=w358, f="" ("Cmd Status")) -> (s? t:f=w359:string)
        n233 = local write "Cmd Status"(w359) -> ()
      }
      event "CheckList": Double Click {
        # "Shift clears all"
        # "Update symbols on the listbox"
        n234 = event-data() -> ("PlatMods.Shift"=w372:bool, "Row"=w374:i32)  [unwired: 1 in]
        n235 = case shown="True" w372 {
          tunnel: w374 -> [w378 _]
          tunnel: 1 -> [w377 _]
          frame False {
            n236 = property on="CheckList" class="LstBox (strict)"() -> ("Item Symbols"=w376:i32[])  [unwired: 2 in, 2 out]
            n237 = Replace Array Subset(array=w376, new element=w377, index=w378) -> (w375:i32[])
            n238 = property on="CheckList" class="LstBox (strict)"("Item Symbols"=w375) -> ()  [unwired: 2 in, 2 out]
          }
          frame True {
            w379 = 0 ("Top Row")
            n239 = property on="CheckList" class="LstBox (strict)"() -> ("Number of Rows"=w381:u32)  [unwired: 2 in, 2 out]
            n240 = Initialize Array(0, w381) -> (w380:i32[])
            n241 = property on="CheckList" class="LstBox (strict)"("Top Row"=w379, "Value"=w379, "Item Symbols"=w380) -> ()  [unwired: 2 in, 2 out]
          }
        }
      }
      event "CheckList": Key Down {
        # "Update symbols on the listbox\nLeft and right keys check and uncheck"
        n242 = event-data() -> ("VKey"=w386:T22)  [unwired: 1 in]
        n243 = case shown="\"Left\", \"Right\"" w386 {
          selector: w386 -> [w391 _]
          tunnel: eventvkey."Left" ("VKey") -> [w389 _]
          frame "Left", "Right" {
            n244 = Equal?(x=w389, y=w391) -> (x = y?=w390:bool)
            n245 = Select(t=0, s=w390, f=1) -> (s? t:f=w392:i32)
            n246 = property on="CheckList" class="LstBox (strict)"() -> ("Item Symbols"=w395:i32[])  [unwired: 2 in, 2 out]
            n247 = Replace Array Subset(array=w395, new element=w392, index="CheckList") -> (w394:i32[])
            n248 = property on="CheckList" class="LstBox (strict)"("Item Symbols"=w394) -> ()  [unwired: 2 in, 2 out]
          }
          frame Default {
          }
        }
      }
      event "DB Camera Config": Value Change {
        # "Show or hide the cluster of controls, store in ini file"
        n249 = event-data() -> ("NewVal"=w400:bool)  [unwired: 1 in]
        n250 = case shown="False" w400 {
          tunnel: w399 -> [w409 _]
          tunnel: [w402 w420] -> w398
          tunnel: w397 -> [w401 w420]
          frame False {
            w416 = "Camera"
            w419 = FALSE ("Visible")
            n251 = local read "Camera Settings"() -> (w408:T2)
            n252 = Index Array(array=w409) -> (element=w412:cluster{string[]})  [unwired: 1 in]
            n253 = Unbundle(w408) -> ("Frame Rate"=w407:i32, "Compression"=w406:i32, "Size"=w410:u16)
            n254 = Unbundle(w412) -> (w411:string[])
            n255 = Index Array(array=w411, index=w410) -> (element=w405:string)
            n256 = call-poly <vilib>:"Write Key.vi"("section"=w416, "value"=w405, "key"="Size", "refnum"=w401) -> ("refnum out"=w418:T20)  [unwired: 2 in, 5 out]
            n257 = call-poly <vilib>:"Write Key.vi"("section"=w416, "value"=w407, "key"="FrameRate", "refnum"=w418) -> ("refnum out"=w417:T20)  [unwired: 1 in, 6 out]
            n258 = property on="Camera Settings" class="Clust (strict)"("Visible"=w419) -> ()  [unwired: 2 in, 2 out]
            n259 = local write "DB Camera Config"(w419) -> ()
            n260 = call-poly <vilib>:"Write Key.vi"("section"=w416, "value"=w406, "key"="Compression", "refnum"=w417) -> ("refnum out"=w403:T20)  [unwired: 1 in, 6 out]
            n261 = call <vilib>:"Close Config Data.vi"("refnum"=w403) -> ("file path"=w404:path)  [unwired: 2 in, 8 out]
            n262 = call <vilib>:"Open Config Data.vi"("configuration file path"=w404) -> ("refnum"=w402:T20)  [unwired: 8 in, 2 out]
          }
          frame True {
            n263 = property on="Camera Settings" class="Clust (strict)"("Visible"=TRUE) -> ()  [unwired: 2 in, 2 out]
          }
        }
      }
      event "Camera Settings": Value Change {
        # "Update summary string when any elements of DB camera change"
        n264 = event-data() -> ("NewVal"=w434:T2)  [unwired: 1 in]
        n265 = Index Array(array=w430) -> (element=w429:cluster{string[]})  [unwired: 1 in]
        n266 = Unbundle(w434) -> ("Frame Rate"=w425:i32, "Compression"=w424:i32, "Size"=w427:u16)
        n267 = Unbundle(w429) -> (w428:string[])
        n268 = Index Array(array=w428, index=w427) -> (element=w426:string)
        n269 = Format Into String(format string="%s   %dfps   %d%%", w426, w425, w424) -> (resulting string=w431:string)  [unwired: 2 in, 1 out]
        n270 = Build Array(w431) -> (w432:string[])
        n271 = property on="DB Camera Config" class="Bool (strict)"("Strings [4]"=w432) -> ()  [unwired: 2 in, 2 out]
      }
      event "Motor.Enable": Value Change {
        # "When the test mode otor enable helper is set, update that\ntree row item's value"
        n272 = event-data() -> ("NewVal"=w441:bool)  [unwired: 1 in]
        n273 = Unbundle("Motor") -> ("Value"=w440:dbl)  [unwired: 1 out]
        n274 = Select(t=w440, s=w441, f=0.0) -> (s? t:f=w438:dbl)
        n275 = call <vilib>:"NT Write Number.vi"("Numeric"=w438, "Name"=w437) -> ()  [unwired: 9 in, 1 out]
      }
      event "Test Slider": Value Change {
        # "When the test mode slider helper is set, update that\ntree row item's value"
        n276 = event-data() -> ("NewVal"=w445:dbl)  [unwired: 1 in]
        n277 = call <vilib>:"NT Write Number.vi"("Numeric"=w445, "Name"=w446) -> ()  [unwired: 9 in, 1 out]
      }
      event "On/Off": Value Change {
        # "When the test mode on/off helper value is set, update that\ntree row item's value"
        n278 = event-data() -> ("NewVal"=w451:bool)  [unwired: 1 in]
        n279 = Boolean To (0,1)(Boolean=w451) -> (0, 1=w450:i16)
        n280 = call <vilib>:"NT Write Number.vi"("Numeric"=w450, "Name"=w449) -> ()  [unwired: 9 in, 1 out]
      }
      event "Rev/Fwd": Value Change {
        # "When the test mode helper value for relays is set, update that\ntree row item's value"
        n281 = event-data() -> ("NewVal.Forward"=w460:bool, "NewVal.Reverse"=w459:bool)  [unwired: 1 in]
        n282 = Boolean To (0,1)(Boolean=w460) -> (0, 1=w456:i16)
        n283 = Boolean To (0,1)(Boolean=w459) -> (0, 1=w458:i16)
        n284 = Negate(x=w458) -> (-x=w457:i16)
        n285 = Add(x=w456, y=w457) -> (x+y=w455:i16)
        n286 = call <vilib>:"NT Write Number.vi"("Numeric"=w455, "Name"=w454) -> ()  [unwired: 9 in, 1 out]
      }
      event "Test Ring": Value Change {
        # "When a test mode helper value is selected from the ring,\nset the tree item's variable to the string value"
        n287 = event-data() -> ("NewVal"=w465:u16)  [unwired: 1 in]
        n288 = property on="Test Ring" class="Ring (strict)"() -> ("Strings []"=w466:string[])  [unwired: 2 in, 2 out]
        n289 = Index Array(array=w466, index=w465) -> (element=w464:string)
        n290 = call <vilib>:"NT Write String.vi"("String"=w464, "Name"=w463) -> ()  [unwired: 9 in, 1 out]
      }
      event "Rec Mode": Value Change {
        # "Update globals for recording mode and path to read log from.\nClear when logging and let NetworkTables set path for vision to\nuse."
        n291 = event-data() -> ("NewVal"=w478:enum32{"Stop", "Record", "Playback"})  [unwired: 1 in]
        n292 = global write "WPI_DashboardLogging Global.vi" "Logging Filename"(path "") -> ()
        n293 = global write "WPI_DashboardLogging Global.vi" "Recording"(w478) -> ()
        n294 = case shown="\"Playback\"" w478 {
          tunnel: w477 -> [_ w480 w489]
          tunnel: [_ _ w488] -> w474
          tunnel: [_ _ w487] -> _
          tunnel: w472 -> [_ _ w485]
          tunnel: cluster{i32, i32} {-250, 170} -> [_ _ w484]
          tunnel: [_ _ T23 {"Image Size"=TRUE, "Image Type"=TRUE, "Pixel Value"=TRUE, "ROI Information"=TRUE, "Zoom Factor"=FALSE} ("Image Information Shown:All Elements")] -> w470
          tunnel: [_ _ TRUE ("Zoom Factor")] -> w469
          tunnel: w468 -> [_ _ w481]
          frame Default {
          }
          frame "Stop", "Record" {
            # "Place Window too"
            n295 = invoke class="VI" method="FP.Close"(reference=w480) -> (reference out=w479:refnum<vi>)  [unwired: 2 in, 2 out]
            n296 = invoke class="VI" method="Abort VI"(reference=w479) -> ()  [unwired: 2 in, 3 out]
          }
          frame "Playback" {
            n297 = call "Open Playback Panel.vi"("Offset"=w484, "DB VI Ref"=w485, "Playback in"=w489) -> ("Playback out"=w486:refnum<vi>)  [unwired: 8 in]
            n298 = register-events(w486, w481) -> (reference out=w488:refnum<event-registration>, error out=w487:errorcluster)  [unwired: 2 in]
          }
        }
        n299 = property on="Camera Image" class="ImageControl"("Image Information Shown"=w470, "Image Information Visible"=w469) -> ()  [unwired: 2 in, 2 out]
        n300 = call <vilib>:"WPI_DashboardNT Log FieldName Cache.vi"("Operation"=enum16{"Lookup/Add", "Index", "Clear"}."Clear") -> ()  [unwired: 8 in, 3 out]
      }
      event Panel Close {
        w491 = enum32{"Stop", "Record", "Playback"}."Stop" ("Rec Mode")
        # "Playback window has been closed, abort"
        n301 = event-data() -> ()  [unwired: 1 in, 4 out]
        n302 = local write "Rec Mode"(w491) -> ()
        n303 = global write "WPI_DashboardLogging Global.vi" "Recording"(w491) -> ()
      }
      event Panel Close {
        # "Abort playback window and ourself"
        n304 = event-data() -> ()  [unwired: 1 in, 4 out]
        n305 = invoke class="VI" method="FP.Close"(reference=w497) -> (reference out=w496:refnum<vi>)  [unwired: 2 in, 2 out]
        n306 = invoke class="VI" method="Abort VI"(reference=w496) -> (error out=w495:errorcluster)  [unwired: 2 in, 2 out]
        n307 = invoke class="VI" method="Abort VI"(error in=w495) -> ()  [unwired: 2 in, 3 out]
      }
      event User Event {
        n308 = event-data() -> ("IDs"=w505:cluster{"RPC field ID":u16, "Unique ID":u16}, "String"=w504:string)  [unwired: 1 in]
        n309 = Bundle("IDs"=w505, "String"=w504) -> (w503:T9)  [unwired: 1 in]
        n310 = call <vilib>:"Retrieve RPC Response.vi"("RPC Response"=w503) -> ("Output"=w500:string[][])  [unwired: 10 in]
        n311 = Build Array (concatenate)(w498, w500) -> (w499:string[][])
        n312 = local write "Command Params"(w499) -> ()
        n313 = local write "Cmd Status"("" ("Cmd Status")) -> ()
      }
      event "Vision": Value Change {
        # "Enable/Disable Compression slider.\nHW USB is hard-coded into the camera"
        n314 = event-data() -> ("NewVal"=w512:u16)  [unwired: 1 in]
        n315 = Equal?(x=w512, y=u32 2 ("milliseconds to wait")) -> (x = y?=w510:bool)
        n316 = Select(t=T24."Disabled and Grayed Out" ("Disabled"), s=w510, f=T24."Enabled" ("Disabled")) -> (s? t:f=w507:T24)
        n317 = property on="Compression" class="Slide (strict)"("DisabledEnum"=w507) -> ()  [unwired: 2 in, 2 out]
      }
      event "Tree": Double Click {
        n318 = event-data() -> ("PlatMods"=w517:T27, "Tag"=w516:string)  [unwired: 1 in]
        n319 = Unbundle(w517) -> ("Shift"=w515:bool)  [unwired: 4 out]
        n320 = Not(x=w515) -> (.not. x?=w514:bool)
        n321 = call <vilib>:"NT Update Persistence.vi"("Persistence"=w514, "Name"=w516) -> ()  [unwired: 9 in, 1 out]
      }
    }
  }
  n322 = while {
    tunnel: w47 -> [w521]
    i -> [w524]
    stop <- FALSE stop-if-true
    n323 = Wait (ms)(milliseconds to wait=u32 100) -> ()  [unwired: 1 out]
    n324 = case shown="\"Playback\"" "Rec Mode" {
      tunnel: w524 -> [_ _ w539]
      tunnel: [u32 2829099 ("Base Color") u32 11141120 ("Target Color") w528] -> w520
      frame "Stop", Default {
        # "Reset the color, extra updates don't cost much"
      }
      frame "Record" {
      }
      frame "Playback" {
        # "Playback"
        n325 = Quotient & Remainder(x=w539, y=u32 50 ("milliseconds to wait")) -> (x-y*floor(x/y)=w535:u32)  [unwired: 1 out]
        n326 = Divide(x=w535, y=u32 50 ("milliseconds to wait")) -> (x/y=w532:dbl)
        n327 = Multiply(x=6.283185307179586, y=w532) -> (x*y=w537:dbl)
        n328 = Sine(x=w537) -> (sin(x)=w536:dbl)
        n329 = Absolute Value(x=w536) -> (abs(x)=w529:dbl)
        n330 = call "Interpolate RGB Color.vi"("Proportion"=w529, "Target Color"=u32 30976, "Base Color"=u32 2829099) -> ("Result Color"=w528:u32)  [unwired: 8 in]
      }
    }
    n331 = property class="Pane"(reference=w521, "PaneColor"=w520) -> ()  [unwired: 1 in, 2 out]
  }
  n332 = local write "Dashboard Tab"(T1."Drive" ("Dashboard Tab")) -> ()
  n333 = property on="On/Off" class="Bool (strict)"("Visible"=w15) -> ()  [unwired: 2 in, 2 out]
  n334 = property on="Motor" class="Clust (strict)"("Visible"=w15) -> ()  [unwired: 2 in, 2 out]
  n335 = property on="Progress" class="Clust (strict)"("Visible"=w15) -> ()  [unwired: 2 in, 2 out]
  n336 = property on="Test Ring" class="Ring (strict)"("Visible"=w15) -> ()  [unwired: 2 in, 2 out]
  n337 = property on="Rev/Fwd" class="Clust (strict)"("Visible"=w15) -> ()  [unwired: 2 in, 2 out]
  n338 = property on="Camera Settings" class="Clust (strict)"("Visible"=w15) -> ()  [unwired: 2 in, 2 out]
  n339 = while {
    tunnel: u16 1741 ("timeout ms (25000)") -> [w541]
    stop <- FALSE stop-if-true
    n340 = TCP Create Listener(10:w541) -> (0:w540:errorcluster, 3:w542:refnum<k5>)  [unwired: 4 in, 1 out]
    n341 = case shown="No Error" w540 {
      selector: w540 -> [w544 _]
      tunnel: w542 -> [w545 _]
      frame No Error {
        n342 = while {
          tunnel: w545 -> [w548]
          tunnel: w544 -> [w547]
          stop <- FALSE stop-if-true
          n343 = TCP Wait On Listener(8:w547, 11:w548) -> (0:w549:errorcluster, 4:w550:refnum<k5>)  [unwired: 2 in, 3 out]
          n344 = local write "TCP"(w550) -> ()
          n345 = case shown="No Error" w549 {
            frame No Error {
            }
            frame Error {
              n346 = Wait (ms)(milliseconds to wait=u32 1000) -> ()  [unwired: 1 out]
            }
          }
        }
      }
      frame Error {
        n347 = Wait (ms)(milliseconds to wait=u32 1000) -> ()  [unwired: 1 out]
      }
    }
  }
  n348 = local write "DB Camera Config"(w15) -> ()
  n349 = local write "Command Params"(string[][] [] ("Command Params")) -> ()
  n350 = global write "WPI_DashboardLogging Global.vi" "Recording"(w41) -> ()
  n351 = local write "Rec Mode"(w41) -> ()
  n352 = local write "Command Selection"(u16 0 ("milliseconds to wait")) -> ()
